vi "2P_AdapUprite_Linlin.vi"() -> ()   [LabVIEW 2015] (continued)
                                n488 = Index Array(array=w2975, index=w2972) -> (element=w2971:T21)
                                }
                                frame #1 {
                                w2989 = 0.0 ("padding value")
                                n489 = call "2pparameters.vi"("command"="get") -> ("params out"=w2987:T12)  [unwired: 1 in]
                                n490 = Unbundle By Name(w2987) -> ("srate"=w2985:sgl, "sAOxy"=w2986:i32)
                                n491 = To Double Precision Float(number=w2985) -> (double precision float=w2983:dbl)
                                n492 = To Double Precision Float(number=w2985) -> (double precision float=w2984:dbl)
                                n493 = To Double Precision Float(number=w2986) -> (double precision float=w2979:dbl)
                                n494 = Divide(x=1.0 ("Digital DC (%)"), y=w2979) -> (x/y=w2978:dbl)
                                n495 = Multiply(x=100.0, y=w2978) -> (x*y=w2977:dbl)
                                n496 = Divide(x=w2984, y=w2979) -> (x/y=w2982:dbl)
                                n497 = call "replace DO wf param.vi"("Digital Freq (Hz)"=w2982, "Digital DC (%)"=w2977, "Digital phase"=w2989, "Sampling frequency (Hz)"=w2983, "Digital time offset (s)"=w2989, "index of DO wave"=w2981, "padding value"=w2989, "matlab wave file"=path "LT" ("matlab wave number")) -> ()  [unwired: 3 in]
                                }
                                }
                                }
                                }
                                n498 = Build Array(w2965) -> (w2964:T20)
                                }
                                }
                              }
                              frame #9 {
                                # "Add lifetime timestamp waveform"
                                n499 = Build Array(w2994, w2993) -> (w2996:bool[])
                                n500 = Boolean Array To Number(Boolean array=w2996) -> (number=w2995:u32)
                                n501 = case shown="2" w2995 {
                                tunnel: w2992 -> [_ w3048 _ w3052]
                                tunnel: [_ w3043 _ w3049] -> w2991
                                frame 1 {
                                n502 = call "2pparameters.vi"("command"="get") -> ("params out"=w3003:T12)  [unwired: 1 in]
                                n503 = Unbundle By Name(w3003) -> ("wavdet"=w3004:bool, "sAOxy"=w3006:i32, "refwfsize"=w3007:dbl, "srate Img"=w3005:sgl)
                                n504 = call "waveformsDObuffer.vi"("command"="get") -> ("DO wf out"=w2999:digitalwaveform[])  [unwired: 1 in]
                                n505 = case shown="True" w3004 {
                                tunnel: [w3011 w3024] -> w3001
                                tunnel: w3005 -> [w3020 w3039]
                                tunnel: w3006 -> [w3010 w3030]
                                tunnel: w3007 -> [_ w3036]
                                frame False {
                                w3014 = u16 0 items=["unsigned binary", "offset binary", "2's complement"] ("data format (offset binary)")
                                n506 = Initialize Array(sgl 0.0, w3010) -> (w3017:sgl[])
                                n507 = Replace Array Subset(array=w3017, new element=sgl 1.0, index=0) -> (w3015:sgl[])
                                n508 = Reciprocal(x=w3020) -> (1/x=w3021:sgl)
                                n509 = Bundle By Name("Y"=w3015, "dt"=w3021) -> (w3012:waveform(sgl))  [unwired: 1 in]
                                n510 = call-poly <vilib>:"Analog to Digital.vi"("data format (offset binary)"=w3014, "compress digital (T)"=TRUE, "full-scale range (pk-pk)"=1.0, "resolution (16 bit)"=1, "analog waveform"=w3012) -> ("digital waveform"=w3011:digitalwaveform)  [unwired: 3 in, 3 out]
                                }
                                frame True {
                                w3027 = u16 0 items=["unsigned binary", "offset binary", "2's complement"] ("data format (offset binary)")
                                n511 = To Double Precision Float(number=w3030) -> (double precision float=w3037:dbl)
                                n512 = Initialize Array(sgl 0.0, w3030) -> (w3032:sgl[])
                                n513 = Divide(x=w3036, y=w3037) -> (x/y=w3034:dbl)
                                n514 = Round Toward +Infinity(x=w3034) -> (ceil(x): smallest int >= x=w3035:dbl)
                                n515 = Replace Array Subset(array=w3032, new element=sgl 1.0, index=0) -> (w3029:sgl[])
                                n516 = for {
                                N: w3035 -> [_]
                                tunnel: w3029 -> [w3041]
                                tunnel: [w3041] -> w3038 mode=concatenating
                                }
                                n517 = Reciprocal(x=w3039) -> (1/x=w3040:sgl)
                                n518 = Bundle By Name("Y"=w3038, "dt"=w3040) -> (w3025:waveform(sgl))  [unwired: 1 in]
                                n519 = call-poly <vilib>:"Analog to Digital.vi"("data format (offset binary)"=w3027, "compress digital (T)"=TRUE, "full-scale range (pk-pk)"=1.0, "resolution (16 bit)"=1, "analog waveform"=w3025) -> ("digital waveform"=w3024:digitalwaveform)  [unwired: 3 in, 3 out]
                                }
                                }
                                n520 = Build Array (concatenate)(w2999, w3001) -> (w2997:digitalwaveform[])
                                n521 = call "waveformsDObuffer.vi"("DO wf in"=w2997, "command"="set") -> ()  [unwired: 1 out]
                                }
                                frame 2 {
                                n522 = call "waveformsDObuffer.vi"("command"="get") -> ("DO wf out"=w3045:digitalwaveform[])  [unwired: 1 in]
                                n523 = Delete From Array(array=w3045, length=1, index=w3048) -> (deleted portion=w3043:digitalwaveform[], array with subset deleted=w3042:digitalwaveform[])
                                n524 = call "waveformsDObuffer.vi"("DO wf in"=w3042, "command"="set") -> ()  [unwired: 1 out]
                                }
                                frame 3, Default {
                                }
                                frame 0 {
                                n525 = local read "Measurement"() -> (w3051:T4)
                                n526 = To Unsigned Long Integer(number=w3051) -> (unsigned 32bit integer=w3050:u32)
                                n527 = case shown="5..7" w3050 {
                                tunnel: w3052 -> [_ w3055]
                                tunnel: [_ w3054] -> w3049
                                frame 0..4, Default {
                                }
                                frame 5..7 {
                                n528 = call "2pparameters.vi"("command"="get") -> ("params out"=w3062:T12)  [unwired: 1 in]
                                n529 = Unbundle By Name(w3062) -> ("wavdet"=w3063:bool, "sAOxy"=w3065:i32, "refwfsize"=w3066:dbl, "srate Img"=w3064:sgl)
                                n530 = call "waveformsDObuffer.vi"("command"="get") -> ("DO wf out"=w3056:digitalwaveform[])  [unwired: 1 in]
                                n531 = Index Array(array=w3056, index=w3055) -> (element=w3057:digitalwaveform)
                                n532 = case shown="True" w3063 {
                                tunnel: [w3070 w3083] -> w3060
                                tunnel: w3064 -> [w3079 w3098]
                                tunnel: w3065 -> [w3069 w3089]
                                tunnel: w3066 -> [_ w3095]
                                frame False {
                                w3073 = u16 0 items=["unsigned binary", "offset binary", "2's complement"] ("data format (offset binary)")
                                n533 = Initialize Array(sgl 0.0, w3069) -> (w3076:sgl[])
                                n534 = Replace Array Subset(array=w3076, new element=sgl 1.0, index=0) -> (w3074:sgl[])
                                n535 = Reciprocal(x=w3079) -> (1/x=w3080:sgl)
                                n536 = Bundle By Name("Y"=w3074, "dt"=w3080) -> (w3071:waveform(sgl))  [unwired: 1 in]
                                n537 = call-poly <vilib>:"Analog to Digital.vi"("data format (offset binary)"=w3073, "compress digital (T)"=TRUE, "full-scale range (pk-pk)"=1.0, "resolution (16 bit)"=1, "analog waveform"=w3071) -> ("digital waveform"=w3070:digitalwaveform)  [unwired: 3 in, 3 out]
                                }
                                frame True {
                                w3086 = u16 0 items=["unsigned binary", "offset binary", "2's complement"] ("data format (offset binary)")
                                n538 = To Double Precision Float(number=w3089) -> (double precision float=w3096:dbl)
                                n539 = Initialize Array(sgl 0.0, w3089) -> (w3091:sgl[])
                                n540 = Divide(x=w3095, y=w3096) -> (x/y=w3093:dbl)
                                n541 = Round Toward +Infinity(x=w3093) -> (ceil(x): smallest int >= x=w3094:dbl)
                                n542 = Replace Array Subset(array=w3091, new element=sgl 1.0, index=0) -> (w3088:sgl[])
                                n543 = for {
                                N: w3094 -> [_]
                                tunnel: w3088 -> [w3100]
                                tunnel: [w3100] -> w3097 mode=concatenating
                                }
                                n544 = Reciprocal(x=w3098) -> (1/x=w3099:sgl)
                                n545 = Bundle By Name("Y"=w3097, "dt"=w3099) -> (w3084:waveform(sgl))  [unwired: 1 in]
                                n546 = call-poly <vilib>:"Analog to Digital.vi"("data format (offset binary)"=w3086, "compress digital (T)"=TRUE, "full-scale range (pk-pk)"=1.0, "resolution (16 bit)"=1, "analog waveform"=w3084) -> ("digital waveform"=w3083:digitalwaveform)  [unwired: 3 in, 3 out]
                                }
                                }
                                n547 = Build Array(w3057) -> (w3054:digitalwaveform[])
                                n548 = Replace Array Subset(array=w3056, new element=w3060, index=w3055) -> (w3053:digitalwaveform[])
                                n549 = call "waveformsDObuffer.vi"("DO wf in"=w3053, "command"="set") -> ()  [unwired: 1 out]
                                }
                                }
                                }
                                }
                              }
                              frame #10 {
                                # "Could this be the source of error?"
                                # "Check that all the waveforms are the right size so it doesn't crash\npossibly resamples all of the waveforms in case the sampling rate changed at some point"
                                n550 = local read "Meastab"() -> (w3115:enum32{"X-Y Image", "Linescan", "Timetrace"})
                                n551 = property on="refwf" class="Ring (strict)"() -> ("RingText.Text"=w3112:string)  [unwired: 2 in, 2 out]
                                n552 = case shown="\"Timetrace\"" w3115 {
                                tunnel: [w3117 w3118] -> w3116
                                frame "X-Y Image", Default {
                                n553 = local read "Sampling rate"() -> (w3117:dbl)
                                }
                                frame "Timetrace" {
                                n554 = local read "srateAODOtt"() -> (w3118:dbl)
                                }
                                }
                                n555 = call "waveformsAObuffer.vi"("command"="get") -> ("AO wf out"=w3103:waveform(dbl)[])  [unwired: 1 in]
                                n556 = local read "wavdet"() -> (w3113:bool)
                                n557 = call "waveformsDObuffer.vi"("command"="get") -> ("DO wf out"=w3107:digitalwaveform[])  [unwired: 1 in]
                                n558 = call "correctwaveformsizetemp.vi"("new sampling frequency (Hz)"=w3116, "start"=TRUE, "reference waveforms to"=w3112, "Analog waveforms in"=w3103, "stop"=FALSE, "Digital waveforms in"=w3107) -> ("analog wf out"=w3109:waveform(dbl)[], "Digital wf out"=w3111:digitalwaveform[], "measpoints"=w3114:i32)
                                n559 = call "GetNumCamFramesv2.vi"("Digital Waveform Graph"=w3111) -> ("Numeric"=w3110:i32)  [unwired: 10 in]
                                n560 = call "waveformsDObuffer.vi"("DO wf in"=w3111, "command"="set") -> ()  [unwired: 1 out]
                                n561 = call "waveformsAObuffer.vi"("AO wf in"=w3109, "command"="set") -> ()  [unwired: 1 out]
                                n562 = local write "Total Camera Frames"(w3110) -> ()
                                n563 = case shown="True" w3113 {
                                tunnel: w3114 -> [_ w3119]
                                frame False {
                                }
                                frame True {
                                n564 = local write "# of frames"(w3119) -> ()
                                }
                                }
                              }
                            }
                          }
                          frame #6 {
                            # "Disabled for conversion to 64 bit"
                            n565 = disable-structure shown="Disabled" {
                              frame Disabled {
                                n566 = local read "Measurement"() -> (w3124:T4)
                                n567 = case shown="\"Lifetime (scan)\"" w3124 {
                                frame "X-Y-t movie", Default {
                                }
                                frame "Lifetime (scan)" {
                                # "total acquisition time"
                                n568 = call "2pparameters.vi"("command"="get") -> ("params out"=w3130:T12)  [unwired: 1 in]
                                n569 = Unbundle By Name(w3130) -> ("measpoints"=w3151:i32, "avpp"=w3152:i32, "sAOxy"=w3131:i32, "srate Img"=w3153:sgl)
                                n570 = Multiply(x=w3151, y=w3152) -> (x*y=w3149:i32)
                                n571 = To Double Precision Float(number=w3131) -> (double precision float=w3136:dbl)
                                n572 = Divide(x=w3136, y=w3153) -> (x/y=w3138:dbl)
                                n573 = To Double Precision Float(number=w3149) -> (double precision float=w3134:dbl)
                                n574 = local read "min phot"() -> (w3145:u32)
                                n575 = local read "expected c/s"() -> (w3146:dbl)
                                n576 = Multiply(x=w3134, y=w3138) -> (x*y=w3132:dbl)
                                n577 = Multiply(x=w3132, y=1000.0) -> (x*y=w3137:dbl)
                                n578 = local read "truncate"() -> (w3144:u32)
                                n579 = To Long Integer(number=w3137) -> (32bit integer=w3147:i32)
                                n580 = To Long Integer(number=w3146) -> (32bit integer=w3148:i32)
                                n581 = local read "Number of Bins"() -> (w3139:u32)
                                n582 = local read item#-1() -> (w3143)
                                n583 = local write "Acquisition time"(w3147) -> ()
                                n584 = local read item#-1() -> (w3141)
                                n585 = local read item#-1() -> (w3142)
                                n586 = local read item#-1() -> (w3140)
                                n587 = call "lifetimeparameters.vi"("command"="get") -> ("Params out"=w3128:T22)  [unwired: 1 in]
                                n588 = Add(x=10, y=w3147) -> (x+y=w3135:i32)
                                n589 = Bundle By Name(cluster=w3128, "acq time"=w3135, "acq rate"=w3148, "# bins"=w3139, "Ch0 Level"=w3140, "Ch1 Level"=w3141, "Ch0 ZeroX"=w3142, "Ch1 ZeroX"=w3143, "min photons"=w3145, "truncate"=w3144) -> (w3127:T22)
                                n590 = local write "Acquisition rate"(w3148) -> ()
                                n591 = call "lifetimeparameters.vi"("Params in"=w3127, "command"="set") -> ()  [unwired: 1 out]
                                }
                                }
                                n592 = local read "min phot"() -> (w3122:u32)
                                n593 = Decrement(x=w3122) -> (x-1=w3123:u32)
                                n594 = To Double Precision Float(number=w3123) -> (double precision float=w3121:dbl)
                                n595 = property on="img_CH1" class="IntGraph (strict)"("ZScale.Minimum"=w3121) -> ()  [unwired: 2 in, 2 out]
                              }
                              frame Enabled {
                              }
                            }
                            n596 = local write "64bit disabled"(TRUE ("64bit disabled")) -> ()
                          }
                          frame #7 {
                            # "Estimate time per frame (to display on front panel)"
                            n597 = local read "Sampling rate"() -> (w3155:dbl)
                            n598 = call "calcdaqtime.vi"("sampling rate"=w3155) -> ("Calc. time per frame (ms)"=w3154:dbl)
                            n599 = local write "Calc. time per frame (ms)"(w3154) -> ()
                          }
                          frame #8 {
                            # "Define 'sample mode' and 'timeout' condition to load into the Clock VI for the DAQ task"
                            n600 = call "2pparameters.vi"("command"="get") -> ("params out"=w3166:T12)  [unwired: 1 in]
                            n601 = local read "Measurement"() -> (w3157:T4)
                            n602 = Unbundle By Name(w3166) -> ("bufferAI"=w3164:i32, "srate"=w3165:sgl)
                            n603 = To Double Precision Float(number=w3164) -> (double precision float=w3158:dbl)
                            n604 = To Double Precision Float(number=w3165) -> (double precision float=w3168:dbl)
                            n605 = case shown="\"X-Y-t movie\", Default" w3157 {
                              tunnel: [w3173 w3177] -> w3156
                              frame "X-Y-t movie", Default {
                                n606 = local read "wavdet"() -> (w3174:bool)
                                n607 = case shown="False" w3174 {
                                tunnel: [w3175 w3176] -> w3173
                                frame False {
                                w3175 = 10123 items=["Finite Samples"=10178, "Continuous Samples"=10123, "Hardware Timed Single Point"=12522] ("sample mode")
                                }
                                frame True {
                                w3176 = 10123 items=["Finite Samples"=10178, "Continuous Samples"=10123, "Hardware Timed Single Point"=12522] ("sample mode")
                                }
                                }
                              }
                              frame "X-Y-Z stack" {
                                w3177 = 10178 items=["Finite Samples"=10178, "Continuous Samples"=10123, "Hardware Timed Single Point"=12522] ("sample mode")
                              }
                            }
                            n608 = Divide(x=w3158, y=w3168) -> (x/y=w3172:dbl)
                            n609 = Multiply(x=w3172, y=2.0) -> (x*y=w3169:dbl)
                            n610 = Max & Min(x=w3169, y=10.0) -> (max(x,y)=w3159:dbl)  [unwired: 1 out]
                            n611 = call "2pparameters.vi"("command"="get") -> ("params out"=w3163:T12)  [unwired: 1 in]
                            n612 = Bundle By Name(cluster=w3163, "timeout"=w3159, "sample mode"=w3156) -> (w3160:T12)
                            n613 = call "2pparameters.vi"("Params in"=w3160, "command"="set") -> ()  [unwired: 1 out]
                          }
                          frame #9 {
                            n614 = local read "# of frames"() -> (w3178:i32)
                            n615 = call "timestamps.vi"("# of frames"=w3178, "command"="init") -> ()  [unwired: 2 in, 1 out]
                          }
                        }
                      }
                      frame #2 {
                        # "Disabled for conversion to 64 bit"
                        n616 = call "prepAO_img.vi"() -> ("Terminal Name with Device Prefix"=w3181:tag)
                        n617 = call "prepAI_img.vi"("triggersource"=w3181) -> ()  [unwired: 2 in]
                        n618 = call "prepCI_img.vi"("ArmStart.DigEdge.Src"=w3181) -> ()  [unwired: 1 in]
                        n619 = call "prepDO_img.vi"() -> ()  [unwired: 2 in]
                        n620 = disable-structure shown="Disabled" {
                          frame Disabled {
                            n621 = local read "Measurement"() -> (w3182:T4)
                            n622 = case shown="\"Lifetime (scan)\"" w3182 {
                              frame "X-Y-t movie", Default {
                              }
                              frame "Lifetime (scan)" {
                                n623 = stacked-sequence {
                                frame #0 {
                                n624 = call "PH-temp.vi"("String"="clear" ("command")) -> ()  [unwired: 2 in, 2 out]
                                n625 = call "PH-temp-raw.vi"("command"="empty") -> ()  [unwired: 1 in, 1 out]
                                }
                                frame #1 {
                                n626 = call "calib.vi"() -> ()  [unwired: 1 in]
                                }
                                frame #2 {
                                n627 = call "setup.vi"() -> ()  [unwired: 1 in]
                                }
                                }
                              }
                            }
                          }
                          frame Enabled {
                          }
                        }
                        n628 = local write "64bit disabled"(TRUE ("64bit disabled")) -> ()
                      }
                      frame #3 {
                        n629 = local read "save\ndata"() -> (w3185:bool)
                        n630 = case shown="True" w3185 {
                          tunnel: w3186 -> [_ w3190]
                          frame False {
                          }
                          frame True {
                            n631 = local read "filename prefix"() -> (w3188:string)
                            n632 = local read "data dir"() -> (w3189:path)
                            n633 = call "preparetiffs_and_headers.vi"("filename prefix"=w3188, "data dir"=w3189, "timestamp"=w3190) -> ("full-filename"=w3187:string)  [unwired: 1 in]
                            n634 = local write "full-filename"(w3187) -> ()
                          }
                        }
                        n635 = call "preptempbuffers.vi"() -> ()  [unwired: 12 in]
                      }
                      frame #4 {
                        # "Go to starting point (in z, if z stack)"
                        # "Disabled Thorlabs Zstage;\nneeds to be replaced by PI code"
                        n636 = local read "Measurement"() -> (w3191:T4)
                        n637 = case shown="\"X-Y-Z stack\"" w3191 {
                          frame "X-Y-t movie", Default {
                          }
                          frame "X-Y-Z stack" {
                            # "Move Z stage"
                            n638 = stacked-sequence {
                              seq-local: [w3194 _] -> [_ w3206]
                              frame #0 {
                                n639 = local read "Z-Start (um)"() -> (w3197:dbl)
                                n640 = local read "Z-end (um)"() -> (w3196:dbl)
                                n641 = local read "# of frames"() -> (w3198:i32)
                                n642 = call "calcZslice.vi"("current slice"=0, "# of Slices"=w3198, "Z-Start (um)"=w3197, "Z-end (um)"=w3196) -> ("zpos (V)"=w3193:dbl, "zpos (um)"=w3194:dbl)
                                n643 = call "moveZ_Sutter.vi"("Z"=w3193) -> ()
                                n644 = local write "Cal. Z"(w3194) -> ()
                              }
                              frame #1 {
                                n645 = local read "Pstart"() -> (w3205:dbl)
                                n646 = local read "Pend"() -> (w3204:dbl)
                                n647 = local read "exp?"() -> (w3203:bool)
                                n648 = local read "Z-Start (um)"() -> (w3208:dbl)
                                n649 = local read "Z0"() -> (w3209:dbl)
                                n650 = local read "Z-end (um)"() -> (w3207:dbl)
                                n651 = local read "wavelength(nm)"() -> (w3202:dbl)
                                n652 = local read "# of frames"() -> (w3201:i32)
                                n653 = call "pockelscellzstage.vi"("current slice"=0, "# of Slices"=w3201, "wavelength (nm)"=w3202, "Z0"=w3209, "exp?"=w3203, "Zstart"=w3208, "Pend"=w3204, "Pstart"=w3205, "Z"=w3206, "Zend"=w3207) -> ("T(%)"=w3199:dbl)  [unwired: 1 in]
                                n654 = property on="Laserpower  (%)" class="Slide (strict)"("Value"=w3199) -> ()  [unwired: 2 in, 2 out]
                                n655 = property on="lpow" class="DigNum (strict)"("Value"=w3199) -> ()  [unwired: 2 in, 2 out]
                              }
                            }
                          }
                        }
                        n656 = local write "Thorlabs Zstage disabled"(TRUE ("64bit disabled")) -> ()
                      }
                      frame #5 {
                        n657 = flat-sequence {
                          frame #0 {
                            n658 = call "2pparameters.vi"("command"="get") -> ("params out"=w3212:T12)  [unwired: 1 in]
                            n659 = Unbundle By Name(w3212) -> ("autoshutter"=w3213:bool, "aAS"=w3210:u32[])
                            n660 = case shown="True" w3213 {
                              tunnel: w3210 -> [_ w3214]
                              frame False {
                              }
                              frame True {
                                n661 = call "shuttercontrol_multi.vi"("Autoshutter Chans"=w3214, "command"="open") -> ()  [unwired: 1 in, 1 out]
                              }
                            }
                          }
                          frame #1 {
                            # "measure position of XYZ stage"
                            n662 = call "getXYZ_Sutter.vi"() -> ("Position in Microns"=w3216:dbl[])
                            "Last Stage Position in Microns" <- w3216
                            n663 = call "2pparameters.vi"("command"="get") -> ("params out"=w3218:T12)  [unwired: 1 in]
                            n664 = Bundle By Name(cluster=w3218, "XYZstart"=w3216) -> (w3217:T12)
                            n665 = call "2pparameters.vi"("Params in"=w3217, "command"="set") -> ()  [unwired: 1 out]
                          }
                          frame #2 {
                            n666 = call "2pparameters.vi"("command"="get") -> ("params out"=w3223:T12)  [unwired: 1 in]
                            n667 = Tick Count (ms)() -> (millisecond timer value=w3222:u32)
                            n668 = Bundle By Name(cluster=w3223, "starttick"=w3222) -> (w3221:T12)
                            n669 = call "2pparameters.vi"("Params in"=w3221, "command"="set") -> ()  [unwired: 1 out]
                          }
                        }
                      }
                      frame #6 {
                        n670 = local read "Measurement"() -> (w3226:T4)
                        n671 = case shown="\"Lifetime (scan)\"" w3226 {
                          frame "X-Y-t movie" {
                            n672 = flat-sequence {
                              frame #0 {
                                n673 = call "runAI_img.vi"() -> ()  [unwired: 12 in]
                                n674 = call "runCI.vi"() -> ()  [unwired: 12 in]
                                n675 = call "runDO_img.vi"() -> ()  [unwired: 12 in]
                              }
                              frame #1 {
                                n676 = call "runAO_img.vi"() -> ()  [unwired: 12 in]
                              }
                            }
                          }
                          frame "Lifetime (scan)" {
                            # "Disabled for conversion to 64 bit"
                            n677 = disable-structure shown="Disabled" {
                              frame Disabled {
                                n678 = flat-sequence {
                                frame #0 {
                                n679 = call "runLT_img.vi"() -> ()  [unwired: 1 in]
                                n680 = call "runDO_img.vi"() -> ()  [unwired: 12 in]
                                }
                                frame #1 {
                                n681 = call "runAI_img.vi"() -> ()  [unwired: 12 in]
                                n682 = call "runCI.vi"() -> ()  [unwired: 12 in]
                                }
                                frame #2 {
                                n683 = call "runAO_img.vi"() -> ()  [unwired: 12 in]
                                }
                                }
                              }
                              frame Enabled {
                              }
                            }
                            n684 = local write "64bit disabled"(TRUE ("64bit disabled")) -> ()
                          }
                          frame "X-Y-Z stack", Default {
                          }
                        }
                      }
                      frame #7 {
                        # "Disabled for conversion to 64 bit"
                        n685 = while {
                          i -> [w3255]
                          stop <- w3252 stop-if-true
                          # "This while loop is for every frame"
                          n686 = local read "Exit"() -> (w3260:bool)
                          n687 = local read "Stop"() -> (w3251:bool)
                          n688 = Or(x=w3251, y=w3260) -> (x .or. y?=w3256:bool)
                          n689 = case shown="False" w3256 {
                            tunnel: w3255 -> [w3261 _]
                            frame False {
                              n690 = stacked-sequence {
                                seq-local: [w3263 _ _ _ _ _ _] -> [_ _ _ _ _ _ w3414]
                                seq-local: [w3262 _ _ _ _ _ _] -> [_ _ _ _ _ _ w3413]
                                tunnel: w3261 -> [_ w3269 _ _ _ _ _]
                                frame #0 {
                                n691 = local read "Live"() -> (w3264:bool)
                                n692 = case shown="True" w3264 {
                                tunnel: [_ w3266] -> w3263
                                tunnel: [_ w3265] -> w3262
                                frame False {
                                }
                                frame True {
                                n693 = local read "Laserpower  (%)"() -> (w3265:dbl)
                                n694 = local read "lpow"() -> (w3266:dbl)
                                }
                                }
                                n695 = call "preptempbuffers.vi"() -> ()  [unwired: 12 in]
                                }
                                frame #1 {
                                # "If XYT movie, monitor stage position here"
                                # "Move in Z if necessary"
                                # "Disabled Thorlabs Zstage;\nneeds to be replaced by PI code"
                                n696 = local read "Measurement"() -> (w3267:T4)
                                n697 = case shown="\"X-Y-t movie\", Default" w3267 {
                                tunnel: w3269 -> [_ w3274]
                                frame "X-Y-t movie", Default {
                                # "This is kind of slow right now, or at least it adds 10s of ms to each frame because it reconnects with the stage after each frame. A faster way would be to maintain connection with the stage during acquisition, but this was the fastest way to code this feature."
                                n698 = case shown="True" "disable slive stage" {
                                tunnel: [dbl[] [] ("Position in Microns") w3273] -> w3270
                                frame False {
                                }
                                frame True {
                                n699 = call "getXYZ_Sutter.vi"() -> ("Position in Microns"=w3273:dbl[])
                                }
                                }
                                "Current frame position in microns" <- w3270
                                }
                                frame "X-Y-Z stack" {
                                # "The Z motion happens below"
                                n700 = stacked-sequence {
                                seq-local: [w3276 _] -> [_ w3283]
                                tunnel: w3274 -> [w3277 w3282]
                                frame #0 {
                                n701 = local read "Z-Start (um)"() -> (w3279:dbl)
                                n702 = local read "Z-end (um)"() -> (w3278:dbl)
                                n703 = local read "# of frames"() -> (w3280:i32)
                                n704 = call "calcZslice.vi"("current slice"=w3277, "# of Slices"=w3280, "Z-Start (um)"=w3279, "Z-end (um)"=w3278) -> ("zpos (V)"=w3275:dbl, "zpos (um)"=w3276:dbl)
                                n705 = local write "Cal. Z"(w3276) -> ()
                                n706 = call "moveZ_Sutter.vi"("Z"=w3275) -> ()
                                }
                                frame #1 {
                                n707 = local read "Pstart"() -> (w3288:dbl)
                                n708 = local read "Pend"() -> (w3287:dbl)
                                n709 = local read "exp?"() -> (w3286:bool)
                                n710 = local read "Z-Start (um)"() -> (w3290:dbl)
                                n711 = local read "Z0"() -> (w3291:dbl)
                                n712 = local read "Z-end (um)"() -> (w3289:dbl)
                                n713 = local read "wavelength(nm)"() -> (w3285:dbl)
                                n714 = local read "# of frames"() -> (w3284:i32)
                                n715 = call "pockelscellzstage.vi"("current slice"=w3282, "# of Slices"=w3284, "wavelength (nm)"=w3285, "Z0"=w3291, "exp?"=w3286, "Zstart"=w3290, "Pend"=w3287, "Pstart"=w3288, "Z"=w3283, "Zend"=w3289) -> ("T(%)"=w3281:dbl)  [unwired: 1 in]
                                n716 = property on="Laserpower  (%)" class="Slide (strict)"("Value"=w3281) -> ()  [unwired: 2 in, 2 out]
                                n717 = property on="lpow" class="DigNum (strict)"("Value"=w3281) -> ()  [unwired: 2 in, 2 out]
                                }
                                }
                                }
                                }
                                n718 = local write "Thorlabs Zstage disabled"(TRUE ("64bit disabled")) -> ()
                                }
                                frame #2 {
                                # "Averaging loop (multiple scans per frame)"
                                # "main loop"
                                n719 = for {
                                N: "avpp" -> [_]
                                i -> [w3297]
                                n720 = local read "Stop"() -> (w3295:bool)
                                n721 = local read "Exit"() -> (w3294:bool)
                                n722 = Increment(x=w3297) -> (x+1=w3296:i32)
                                n723 = Or(x=w3295, y=w3294) -> (x .or. y?=w3293:bool)
                                n724 = case shown="False" w3293 {
                                tunnel: w3296 -> [w3298 _]
                                frame False {
                                n725 = stacked-sequence {
                                seq-local: [w3299 _ _ _ _ _ _] -> [_ _ _ w3314 w3340 w3348 _]
                                tunnel: w3298 -> [w3300 _ _ _ _ _ _]
                                frame #0 {
                                n726 = local read "Live"() -> (w3299:bool)
                                n727 = case shown="True" w3299 {
                                tunnel: w3300 -> [_ w3303]
                                frame False {
                                }
                                frame True {
                                # "collect timetag for current image\nplus curent average"
                                n728 = To Single Precision Float(number=w3303) -> (single precision float=w3301:sgl)
                                n729 = Tick Count (ms)() -> (millisecond timer value=w3302:u32)
                                n730 = local write "Tick for Frame"(w3302) -> ()
                                n731 = local write "Current Average"(w3301) -> ()
                                }
                                }
                                }
                                frame #1 {
                                n732 = local read "Measurement"() -> (w3304:T4)
                                n733 = case shown="\"X-Y-Z stack\"" w3304 {
                                frame "X-Y-t movie", Default {
                                }
                                frame "X-Y-Z stack" {
                                n734 = stacked-sequence {
                                frame #0 {
                                n735 = disable-structure shown="Disabled" {
                                frame Disabled {
                                n736 = call "2pparameters.vi"("command"="get") -> ("params out"=w3307:T12)  [unwired: 1 in]
                                n737 = Unbundle By Name(w3307) -> ("autoshutter"=w3308:bool, "aAS"=w3305:u32[])
                                n738 = case shown="True" w3308 {
                                tunnel: w3305 -> [_ w3309]
                                frame False {
                                }
                                frame True {
                                n739 = call "shuttercontrol_multi.vi"("Autoshutter Chans"=w3309, "command"="open") -> ()  [unwired: 1 in, 1 out]
                                }
                                }
                                }
                                frame Enabled {
                                }
                                }
                                }
                                frame #1 {
                                n740 = call "runAI_img.vi"() -> ()  [unwired: 12 in]
                                n741 = call "runCI.vi"() -> ()  [unwired: 12 in]
                                n742 = call "runDO_img.vi"() -> ()  [unwired: 12 in]
                                }
                                frame #2 {
                                n743 = call "runAO_img.vi"() -> ()  [unwired: 12 in]
                                }
                                }
                                }
                                }
                                }
                                frame #2 {
                                n744 = call "collectCI_img.vi"() -> ("Avg cts/s"=w3313:dbl, "recorded samples"=w3312:i32)  [unwired: 1 out]
                                n745 = call "collectAI_img.vi"() -> ("wrap"=w3311:i32)  [unwired: 3 in]
                                n746 = local write "scol"(w3312) -> ()
                                n747 = local write "wrap"(w3311) -> ()
                                n748 = local write "Avg Counts/s"(w3313) -> ()
                                }
                                frame #3 {
                                n749 = case shown="True" w3314 {
                                frame False {
                                }
                                frame True {
                                n750 = local read "Measurement"() -> (w3315:T4)
                                n751 = case shown="\"X-Y-t movie\", Default" w3315 {
                                frame "X-Y-t movie", Default {
                                n752 = local read "ROI Type"() -> (w3316:u16)
                                n753 = case shown="0" w3316 {
                                frame 0 {
                                # "display chosen channels"
                                n754 = local read "image1list chB"() -> (w3329:u16)
                                n755 = local read "image1list chA"() -> (w3330:u16)
                                n756 = local read "Current Average"() -> (w3331:sgl)
                                n757 = local read "image1list"() -> (w3337:u16)
                                n758 = local read "image2list"() -> (w3334:u16)
                                n759 = To Unsigned Word Integer(number=w3334) -> (unsigned 16bit integer=w3335:u16)
                                n760 = To Unsigned Word Integer(number=w3337) -> (unsigned 16bit integer=w3336:u16)
                                n761 = To Unsigned Word Integer(number=w3329) -> (unsigned 16bit integer=w3333:u16)
                                n762 = To Unsigned Word Integer(number=w3330) -> (unsigned 16bit integer=w3332:u16)
                                n763 = local read "chB_Int"() -> (w3327:dbl)
                                n764 = local read "chA_Int"() -> (w3328:dbl)
                                n765 = local read "Image"() -> (w3323:T6)
                                n766 = call "dattoimage.vi"("image2list"=w3335, "Current Average"=w3331, "image1list"=w3336) -> ("image 2 array out"=w3339:sgl[][], "image 1 array out"=w3338:sgl[][])
                                n767 = call "dattoimage.vi"("image2list"=w3333, "Current Average"=w3331, "image1list"=w3332) -> ("image 2 array out"=w3325:sgl[][], "image 1 array out"=w3326:sgl[][])
                                n768 = Transpose 2D Array(2D array=w3338) -> (transposed array=w3322:sgl[][])
                                n769 = Transpose 2D Array(2D array=w3339) -> (transposed array=w3318:sgl[][])
                                n770 = call "disp_dual.vi"("I_B"=w3327, "I_A"=w3328, "img_CHB"=w3325, "img_CHA"=w3326, "Image Dst"=w3323) -> ("Image"=w3324:T6)  [unwired: 6 in]
                                n771 = local write "Image"(w3324) -> ()
                                n772 = call-poly <userlib>:"Reverse 2D Array__ogtk.vi"("by rows or columns (rows)"=enum16{"rows", "columns"}."columns", "Array"=w3318) -> ("Reversed Array"=w3317:sgl[][])  [unwired: 1 in]
                                n773 = call-poly <userlib>:"Reverse 2D Array__ogtk.vi"("by rows or columns (rows)"=enum16{"rows", "columns"}."columns", "Array"=w3322) -> ("Reversed Array"=w3321:sgl[][])  [unwired: 1 in]
                                n774 = local write "img_CH1"(w3321) -> ()
                                n775 = local write "img_CH2"(w3317) -> ()
                                }
                                frame 1, Default {
                                }
                                }
                                }
                                frame "Lifetime (scan)" {
                                }
                                }
                                }
                                }
                                }
                                frame #4 {
                                n776 = case shown="True" w3340 {
                                frame False {
                                }
                                frame True {
                                # "set colormaps"
                                n777 = call "misc-global.vi"("command"="get") -> ("misc out"=w3344:cluster{"Colormaps":u32[][]})  [unwired: 1 in]
                                n778 = Unbundle By Name(w3344) -> ("Colormaps"=w3343:u32[][])
                                n779 = control-ref of="img_CH1"() -> (w3347:refnum<vi>)
                                n780 = control-ref of="img_CH2"() -> (w3346:refnum<vi>)
                                n781 = Index Array(array=w3343, index (row)="Colormap") -> (element=w3342:u32[])  [unwired: 1 in]
                                n782 = property class="IntGraph (strict)"(reference=w3347, "Color Table"=w3342) -> ()  [unwired: 1 in, 2 out]
                                n783 = property class="IntGraph (strict)"(reference=w3346, "Color Table"=w3342) -> ()  [unwired: 1 in, 2 out]
                                }
                                }
                                }
                                frame #5 {
                                n784 = case shown="True" w3348 {
                                frame False {
                                }
                                frame True {
                                # "crude estimate of time per frame\n(resolution is 1 ms), not so much for\nplotting purposes, more for debugging\ncollection and processing data"
                                n785 = local read "ypixels ref"() -> (w3353:i32)
                                n786 = local read "Tick for Frame"() -> (w3354:u32)
                                n787 = Tick Count (ms)() -> (millisecond timer value=w3355:u32)
                                n788 = To Double Precision Float(number=w3353) -> (double precision float=w3352:dbl)
                                n789 = Subtract(x=w3355, y=w3354) -> (x-y=w3350:u32)
                                n790 = To Double Precision Float(number=w3350) -> (double precision float=w3351:dbl)
                                n791 = Divide(x=w3351, y=w3352) -> (x/y=w3349:dbl)
                                n792 = local write "Meas. ms/frame"(w3350) -> ()
                                n793 = local write "time per line (ms)"(w3349) -> ()
                                }
                                }
                                }
                                frame #6 {
                                n794 = local read "Measurement"() -> (w3356:T4)
                                n795 = case shown="\"X-Y-Z stack\"" w3356 {
                                frame "X-Y-t movie", Default {
                                }
                                frame "X-Y-Z stack" {
                                # "Stop scanning ->\n(In order to be able to make a task to move in Z)"
                                n796 = call "2pparameters.vi"("command"="get") -> ("params out"=w3359:T12)  [unwired: 1 in]
                                n797 = Unbundle By Name(w3359) -> ("autoshutter"=w3360:bool, "aAS"=w3357:u32[])
                                n798 = call "stopCI_img.vi"() -> ()  [unwired: 12 in]
                                n799 = call "stopAI_img.vi"() -> ()  [unwired: 12 in]
                                n800 = case shown="True" w3360 {
                                tunnel: w3357 -> [_ w3362]
                                frame False {
                                }
                                frame True {
                                n801 = call "shuttercontrol_multi.vi"("Autoshutter Chans"=w3362, "command"="close") -> ()  [unwired: 1 in, 1 out]
                                }
                                }
                                n802 = Wait (ms)(milliseconds to wait=u32 100) -> ()  [unwired: 1 out]
                                n803 = call "stopAO_img.vi"() -> ()  [unwired: 12 in]
                                n804 = call "stopDO_img.vi"() -> ()  [unwired: 12 in]
                                }
                                }
                                }
                                }
                                }
                                frame True {
                                }
                                }
                                }
                                }
                                frame #3 {
                                # "Save (possibly averaged) data"
                                n805 = local read "Measurement"() -> (w3364:T4)
                                n806 = case shown="\"X-Y-t movie\", Default" w3364 {
                                frame "X-Y-t movie", Default {
                                }
                                frame "Lifetime (scan)" {
                                w3367 = u16 2 items=["Stream to disk", "Post process", "real time process"] ("Ring")
                                n807 = local read "T3R Data processing"() -> (w3368:u16)
                                n808 = Equal?(x=w3368, y=w3367) -> (x = y?=w3366:bool)
                                n809 = case shown="True" w3366 {
                                frame False {
                                }
                                frame True {
                                n810 = disable-structure shown="Disabled" {
                                frame Disabled {
                                n811 = local read "lineshift"() -> (w3371:i32)
                                n812 = call "wrapcutlifetime.vi"("lineshift"=w3371) -> ("pt3img"=w3373:u16[][], "lifetimes"=w3372:sgl[][], "okay"=w3369:bool, "# of frames"=w3370:i32)
                                n813 = case shown="True" w3369 {
                                tunnel: w3373 -> [_ w3383]
                                tunnel: w3372 -> [_ w3381]
                                tunnel: w3370 -> [_ w3377]
                                frame False {
                                }
                                frame True {
                                # "lifetime"
                                # "intensity"
                                n814 = Transpose 2D Array(2D array=w3383) -> (transposed array=w3375:u16[][])
                                n815 = Transpose 2D Array(2D array=w3381) -> (transposed array=w3382:sgl[][])
                                n816 = local write "frames recorded"(w3377) -> ()
                                n817 = local read "counts"() -> (w3376:i32)
                                n818 = Array Max & Min(array=w3375) -> (max value=w3380:u16)  [unwired: 3 out]
                                n819 = To Single Precision Float(number=w3375) -> (single precision float=w3374:sgl[][])
                                n820 = local write "img_CH2"(w3382) -> ()
                                n821 = local write "img_CH1"(w3374) -> ()
                                n822 = Quotient & Remainder(x=w3376, y=w3377) -> (floor(x/y)=→"photons/frame":i32)  [unwired: 1 out]
                                n823 = To Double Precision Float(number=w3380) -> (double precision float=w3379:dbl)
                                n824 = property on="img_CH1" class="IntGraph (strict)"("ZScale.Maximum"=w3379) -> ()  [unwired: 2 in, 2 out]
                                }
                                }
                                }
                                frame Enabled {
                                }
                                }
                                }
                                }
                                }
                                }
                                n825 = local read "save\ndata"() -> (w3365:bool)
                                n826 = case shown="True" w3365 {
                                frame False {
                                }
                                frame True {
                                n827 = local read "Current Average"() -> (w3384:sgl)
                                n828 = call "savetiffs.vi"("current average"=w3384) -> ()
                                }
                                }
                                }
                                frame #4 {
                                # "Saves a list of timestamps for each frame"
                                n829 = local read "save\ndata"() -> (w3385:bool)
                                n830 = case shown="True" w3385 {
                                frame False {
                                }
                                frame True {
                                n831 = local read "points recorded"() -> (w3387:i32)
                                n832 = call "timestamps.vi"("points recorded"=w3387, "command"="add") -> ()  [unwired: 2 in, 1 out]
                                }
                                }
                                }
                                frame #5 {
                                n833 = local read "Live"() -> (w3388:bool)
                                n834 = case shown="True" w3388 {
                                frame False {
                                }
                                frame True {
                                # "for moving Daan's\nxy stage\n(for during live imaging\nfor example)"
                                n835 = local read "downright"() -> (w3393:bool)
                                n836 = local read "downleft"() -> (w3395:bool)
                                n837 = local read "upright"() -> (w3391:bool)
                                n838 = local read "upleft"() -> (w3389:bool)
                                n839 = local read "down"() -> (w3394:bool)
                                n840 = local read "right"() -> (w3392:bool)
                                n841 = local read "left"() -> (w3396:bool)
                                n842 = local read "up"() -> (w3390:bool)
                                n843 = Compound Arithmetic op=OR(w3389, w3390, w3391, w3392, w3393, w3394, w3395, w3396) -> (w3397:bool)
                                n844 = case shown="True" w3397 {
                                frame False {
                                }
                                frame True {
                                n845 = stacked-sequence {
                                frame #0 {
                                n846 = local read "downright"() -> (w3399:bool)
                                n847 = local read "downleft"() -> (w3401:bool)
                                n848 = local read "BigSmall"() -> (w3398:bool)
                                n849 = local read "upright"() -> (w3403:bool)
                                n850 = local read "upleft"() -> (w3406:bool)
                                n851 = local read "down"() -> (w3402:bool)
                                n852 = local read "right"() -> (w3404:bool)
                                n853 = local read "left"() -> (w3400:bool)
                                n854 = local read "up"() -> (w3405:bool)
                                n855 = call "movestageparams.vi"("command"="get") -> ("Params out"=w3409:T23)  [unwired: 1 in]
                                n856 = Bundle By Name(cluster=w3409, "upleft"=w3406, "up"=w3405, "upright"=w3403, "right"=w3404, "downright"=w3399, "down"=w3402, "downleft"=w3401, "left"=w3400, "Bigsmall"=w3398) -> (w3410:T23)
                                n857 = call "movestageparams.vi"("Params in"=w3410, "command"="set") -> ()  [unwired: 1 out]
                                }
                                frame #1 {
                                n858 = call "movestage.vi"() -> ()  [unwired: 12 in]
                                }
                                frame #2 {
                                w3411 = FALSE ("OK Button")
                                w3412 = FALSE ("OK Button")
                                n859 = property on="down" class="Bool (strict)"("Value"=w3412) -> ()  [unwired: 2 in, 2 out]
                                n860 = property on="up" class="Bool (strict)"("Value"=w3412) -> ()  [unwired: 2 in, 2 out]
                                n861 = property on="right" class="Bool (strict)"("Value"=w3412) -> ()  [unwired: 2 in, 2 out]
                                n862 = property on="left" class="Bool (strict)"("Value"=w3412) -> ()  [unwired: 2 in, 2 out]
                                n863 = property on="upright" class="Bool (strict)"("Value"=w3411) -> ()  [unwired: 2 in, 2 out]
                                n864 = property on="downleft" class="Bool (strict)"("Value"=w3411) -> ()  [unwired: 2 in, 2 out]
                                n865 = property on="downright" class="Bool (strict)"("Value"=w3411) -> ()  [unwired: 2 in, 2 out]
                                n866 = property on="upleft" class="Bool (strict)"("Value"=w3411) -> ()  [unwired: 2 in, 2 out]
                                }
                                }
                                }
                                }
                                }
                                }
                                }
                                frame #6 {
                                n867 = local read "Live"() -> (w3415:bool)
                                n868 = case shown="True" w3415 {
                                tunnel: w3414 -> [_ w3422]
                                tunnel: w3413 -> [_ w3421]
                                frame False {
                                }
                                frame True {
                                # "Changing the pockels cell power from front panel\n\nChekcs the value of the front panel after each frame"
                                n869 = local read "Laserpower  (%)"() -> (w3417:dbl)
                                n870 = local read "lpow"() -> (w3416:dbl)
                                n871 = Not Equal?(x=w3416, y=w3422) -> (x != y?=w3418:bool)
                                n872 = Not Equal?(x=w3417, y=w3421) -> (x != y?=w3419:bool)
                                n873 = Or(x=w3419, y=w3418) -> (x .or. y?=w3420:bool)
                                n874 = case shown="True" w3420 {
                                tunnel: w3419 -> [_ w3426]
                                tunnel: w3418 -> [_ w3425]
                                tunnel: w3417 -> [_ w3424]
                                tunnel: w3416 -> [_ w3423]
                                frame False {
                                }
                                frame True {
                                n875 = case shown="True" w3426 {
                                tunnel: w3424 -> [_ w3429]
                                frame False {
                                }
                                frame True {
                                n876 = local read "wavelength(nm)"() -> (w3430:dbl)
                                n877 = call "setpockelscellT.vi"("wavelength(nm)"=w3430, "transmission"=w3429) -> ()  [unwired: 1 in]
                                n878 = property on="lpow" class="DigNum (strict)"("Value"=w3429) -> ()  [unwired: 2 in, 2 out]
                                }
                                }
                                n879 = case shown="True" w3425 {
                                tunnel: w3423 -> [_ w3427]
                                frame False {
                                }
                                frame True {
                                n880 = local read "wavelength(nm)"() -> (w3428:dbl)
                                n881 = call "setpockelscellT.vi"("wavelength(nm)"=w3428, "transmission"=w3427) -> ()  [unwired: 1 in]
                                n882 = property on="Laserpower  (%)" class="Slide (strict)"("Value"=w3427) -> ()  [unwired: 2 in, 2 out]
                                }
                                }
                                }
                                }
                                }
                                }
                                }
                              }
                            }
                            frame True {
                            }
                          }
                          n883 = Increment(x=w3255) -> (x+1=w3254:i32)
                          "points recorded" <- w3254
                          n884 = call "stopcond.vi"("prec"=w3254) -> ("stop"=w3253:bool)
                          n885 = local read "Stop"() -> (w3259:bool)
                          n886 = local read "Exit"() -> (w3258:bool)
                          n887 = Or(x=w3259, y=w3258) -> (x .or. y?=w3257:bool)
                          n888 = Or(x=w3253, y=w3257) -> (x .or. y?=w3252:bool)
                        }
                        n889 = disable-structure shown="Disabled" {
                          disable-tunnel: w3229 -> [w3235 _]
                          frame Disabled {
                            w3232 = u16 0 items=["Stream to disk", "Post process", "real time process"] ("Ring")
                            n890 = local read "T3R Data processing"() -> (w3231:u16)
                            n891 = Equal?(x=w3231, y=w3232) -> (x = y?=w3230:bool)
                            n892 = local read "save\ndata"() -> (w3234:bool)
                            n893 = local read "Measurement"() -> (w3236:T4)
                            n894 = And(x=w3234, y=w3230) -> (x .and. y?=w3233:bool)
                            n895 = case shown="\"Lifetime (scan)\"" w3236 {
                              tunnel: w3235 -> [_ w3240]
                              tunnel: w3233 -> [_ w3239]
                              frame "X-Y-t movie", Default {
                              }
                              frame "Lifetime (scan)" {
                                n896 = case shown="True" w3239 {
                                selector: w3239 -> [w3241 w3246]
                                tunnel: w3240 -> [_ w3244]
                                tunnel: [path "" ("appended path") w3247] -> w3238
                                tunnel: [w3241 w3246] -> w3237
                                frame False {
                                }
                                frame True {
                                n897 = local read "filename prefix"() -> (w3245:string)
                                n898 = local read "data dir"() -> (w3248:path)
                                n899 = call "generatedatafilename.vi"("timestamp"=w3244, "filename prefix in"=w3245) -> ("full-filename"=w3243:string)
                                n900 = Concatenate Strings(w3243, ".lvpt3img" ("string")) -> (w3250:string)
                                n901 = Build Path(base path=w3248, name or relative path=w3250) -> (appended path=w3247:path)
                                }
                                }
                                n902 = call "collectLT_img_v2.vi"("stream?"=w3237, "data file"=w3238) -> ()  [unwired: 2 out]
                              }
                            }
                          }
                          frame Enabled {
                          }
                        }
                        n903 = local write "64bit disabled"(TRUE ("64bit disabled")) -> ()
                      }
                      frame #8 {
                        # "Disabled for conversion to 64 bit"
                        n904 = local read "Measurement"() -> (w3433:T4)
                        n905 = case shown="\"X-Y-Z stack\"" w3433 {
                          tunnel: w3432 -> [_ _ w3434]
                          frame "X-Y-t movie", Default {
                          }
                          frame "X-Y-Z stack" {
                            n906 = call "eraseDO_img.vi"() -> ()  [unwired: 12 in]
                            n907 = call "eraseAO_img.vi"() -> ()  [unwired: 12 in]
                            n908 = call "eraseCI_img.vi"() -> ()  [unwired: 12 in]
                            n909 = call "eraseAI_img.vi"() -> ()  [unwired: 12 in]
                          }
                          frame "Lifetime (scan)" {
                            n910 = disable-structure shown="Disabled" {
                              disable-tunnel: w3434 -> [w3435 _]
                              frame Disabled {
                                n911 = stacked-sequence {
                                tunnel: w3435 -> [_ _ w3449 _ _]
                                frame #0 {
